vi "FillRectangleForChart.vi"(8 "colorRectangle":u32(colorbox)=16860, 9 "y":i16=50, 10 "x":i16=11, 11 "PictureIn":picture) -> (3 "PictureOut":picture)   [LabVIEW 2014]
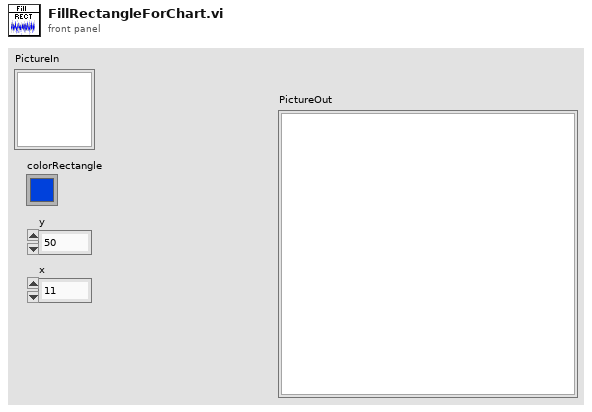
[diagram p1: front panel]
types:
  T1 = cluster{"x":i16, "yOutput":i16, "xOutput":i16, "bottom of rectagle":i16}
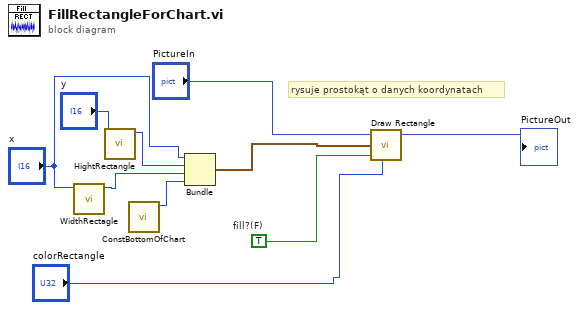
[diagram p0: block diagram]
diagram:
  w10 = TRUE  # fill?(F)
  # "rysuje prostokąt o danych koordynatach"
  n1 = call "WidthRectagle.vi"("xInput"="x") -> ("xOutput"=w4:i16)  [unwired: 10 in]
  n2 = call "HightRectangle.vi"("yInput"="y") -> ("yOutput"=w1:i16)  [unwired: 10 in]
  n3 = call "ConstBottomOfChart.vi"() -> ("bottom of rectagle"=w5:i16)  [unwired: 11 in]
  n4 = Bundle "Bundle"("x"="x", "yOutput"=w1, "xOutput"=w4, "bottom of rectagle"=w5) -> (w9:T1)  [unwired: 1 in]
  n5 = call <vilib>:"Draw Rectangle.vi"("picture"="PictureIn", "rect"=w9, "fill?(F)"=w10, "color(black)"="colorRectangle") -> ("new picture"=→"PictureOut":picture)  [unwired: 5 in]
